vi "HTTP_GET_Test_Arduino_GetData.vi"(11 "reqnum":string) -> (3 "body":string)   [LabVIEW 2017]
panel:
  out "concatenated string":string
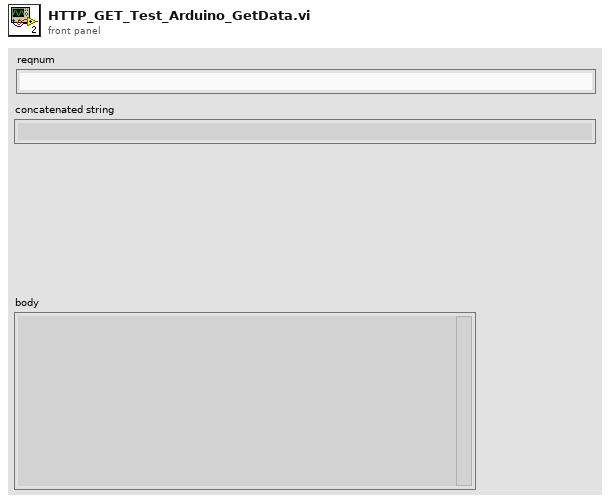
[diagram p1: front panel]
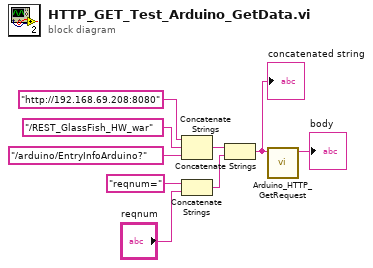
[diagram p0: block diagram]
diagram:
  n1 = Concatenate Strings("http://192.168.69.208:8080" ("url"), "/REST_GlassFish_HW_war" ("url"), "/arduino/EntryInfoArduino?" ("url")) -> (w6:string)
  n2 = Concatenate Strings("reqnum=" ("url"), "reqnum") -> (w5:string)
  n3 = Concatenate Strings(w6, w5) -> (w2:string)
  "concatenated string" <- w2
  n4 = call "Arduino_HTTP_GetRequest.vi"("Request string"=w2) -> ("body"=→"body":string)  [unwired: 10 in]
